vi "PubSubSync.vi"() -> ()   [LabVIEW 2025]
uses:
  libzmq-v143-mt-4_3_6/ctls/SocketType.ctl
  libzmq-v143-mt-4_3_6/ctls/SocketOption.ctl
  zeromq/Receive_string.vi
  zeromq/Send_string.vi
  zeromq/Context.lvclass
  libzmq-v143-mt-4_3_6/LibZMQ.lvlib
  zeromq/Socket.lvclass
panel:
  out "data 2":string
  out "data":string
  out "error out 2":errorcluster
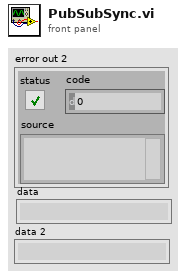
[diagram p1: front panel]
types:
  T1 = typedef "LibZMQ.lvlib/SocketOption.ctl" = enum8{"NONE", "ZMQ_HWM", "<2>", "ZMQ_SWAP", "ZMQ_AFFINITY", "ZMQ_ROUTING_ID", "ZMQ_SUBSCRIBE", "ZMQ_UNSUBSCRIBE", "ZMQ_RATE", "ZMQ_RECOVERY_IVL", "ZMQ_MCAST_LOOP", "ZMQ_SNDBUF", "ZMQ_RCVBUF", "ZMQ_RCVMORE", "ZMQ_FD", "ZMQ_EVENTS", "ZMQ_TYPE", "ZMQ_LINGER", "ZMQ_RECONNECT_IVL", "ZMQ_BACKLOG", "ZMQ_RECOVERY_IVL_MSEC", "ZMQ_RECONNECT_IVL_MAX", "ZMQ_MAXMSGSIZE", "ZMQ_SNDHWM", "ZMQ_RCVHWM", "ZMQ_MULTICAST_HOPS", "<26>", "ZMQ_RCVTIMEO", "ZMQ_SNDTIMEO", "<29>", "<30>", "ZMQ_IPV4ONLY", "ZMQ_LAST_ENDPOINT", "ZMQ_ROUTER_MANDATORY", "ZMQ_TCP_KEEPALIVE", "ZMQ_TCP_KEEPALIVE_CNT", "ZMQ_TCP_KEEPALIVE_IDLE", "ZMQ_TCP_KEEPALIVE_INTVL", "ZMQ_TCP_ACCEPT_FILTER", "ZMQ_IMMEDIATE", "ZMQ_XPUB_VERBOSE", "ZMQ_ROUTER_RAW", "ZMQ_IPV6", "ZMQ_MECHANISM", "ZMQ_PLAIN_SERVER", "ZMQ_PLAIN_USERNAME", "ZMQ_PLAIN_PASSWORD", "ZMQ_CURVE_SERVER", "ZMQ_CURVE_PUBLICKEY", "ZMQ_CURVE_SECRETKEY", "ZMQ_CURVE_SERVERKEY", "ZMQ_PROBE_ROUTER", "ZMQ_REQ_CORRELATE", "ZMQ_REQ_RELAXED", "ZMQ_CONFLATE", "ZMQ_ZAP_DOMAIN", "ZMQ_ROUTER_HANDOVER", "ZMQ_TOS", "ZMQ_IPC_FILTER_PID", "ZMQ_IPC_FILTER_UID", "ZMQ_IPC_FILTER_GID", "ZMQ_CONNECT_ROUTING_ID", "ZMQ_GSSAPI_SERVER", "ZMQ_GSSAPI_PRINCIPAL", "ZMQ_GSSAPI_SERVICE_PRINCIPAL", "ZMQ_GSSAPI_PLAINTEXT", "ZMQ_HANDSHAKE_IVL", "<67>", "ZMQ_SOCKS_PROXY", "ZMQ_XPUB_NODROP", "ZMQ_BLOCKY", "ZMQ_XPUB_MANUAL", "ZMQ_XPUB_WELCOME_MSG", "ZMQ_STREAM_NOTIFY", "ZMQ_INVERT_MATCHING", "ZMQ_HEARTBEAT_IVL", "ZMQ_HEARTBEAT_TTL", "ZMQ_HEARTBEAT_TIMEOUT", "ZMQ_XPUB_VERBOSER", "ZMQ_CONNECT_TIMEOUT", "ZMQ_TCP_MAXRT", "ZMQ_THREAD_SAFE", "<82>", "<83>", "ZMQ_MULTICAST_MAXTPDU", "ZMQ_VMCI_BUFFER_SIZE", "ZMQ_VMCI_BUFFER_MIN_SIZE", "ZMQ_VMCI_BUFFER_MAX_SIZE", "ZMQ_VMCI_CONNECT_TIMEOUT", "ZMQ_USE_FD", "ZMQ_GSSAPI_PRINCIPAL_NAMETYPE", "ZMQ_GSSAPI_SERVICE_PRINCIPAL_NAMETYPE", "ZMQ_BINDTODEVICE", "ZMQ_ZAP_ENFORCE_DOMAIN", "ZMQ_LOOPBACK_FASTPATH", "ZMQ_METADATA", "ZMQ_MULTICAST_LOOP", "ZMQ_ROUTER_NOTIFY"}
  T2 = typedef "LibZMQ.lvlib/SocketType.ctl" = enum8{"PAIR", "PUB", "SUB", "REQ", "REP", "DEALER", "ROUTER", "PULL", "PUSH", "XPUB", "XSUB", "STREAM"}
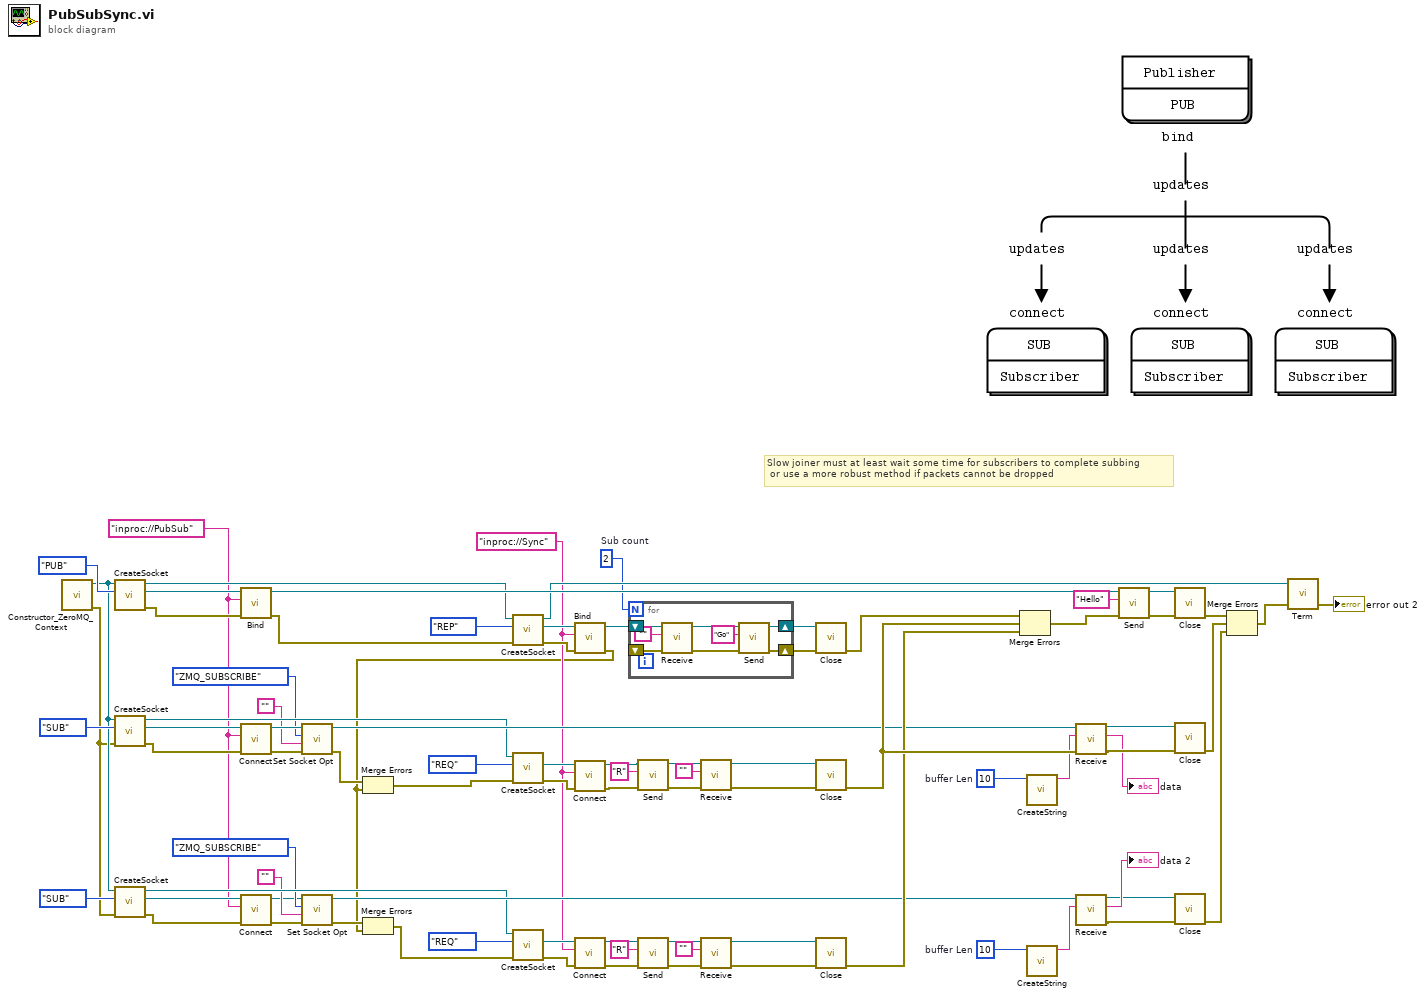
[diagram p0: block diagram]
diagram:
  w1 = "inproc://PubSub"
  w27 = 2  # Sub count
  w41 = "inproc://Sync"
  w61 = 10  # buffer Len
  w71 = 10  # buffer Len
  # "Slow joiner must at least wait some time for subscribers to complete subbing\n or use a more robust method if packets cannot be dropped"
  n1 = call "Constructor_ZeroMQ_Context.vi"() -> ("error out"=w16:errorcluster, "context out"=w57:refnum<class "Context.lvclass">)  [unwired: 10 in]
  n2 = call "CreateSocket.vi"("Socket Type"=SocketType."PUB", "context in"=w57) -> ("error out"=w25:errorcluster, "socket out"=w83:refnum<class "Socket.lvclass">, "context out"=w54:refnum<class "Context.lvclass">)  [unwired: 7 in]
  n3 = call "CreateSocket.vi"("error in"=w16, "Socket Type"=SocketType."SUB", "context in"=w57) -> ("error out"=w24:errorcluster, "socket out"=w81:refnum<class "Socket.lvclass">, "context out"=w46:refnum<class "Context.lvclass">)  [unwired: 6 in]
  n4 = call "CreateSocket.vi"("error in"=w16, "Socket Type"=SocketType."SUB", "context in"=w57) -> ("error out"=w23:errorcluster, "socket out"=w58:refnum<class "Socket.lvclass">, "context out"=w42:refnum<class "Context.lvclass">)  [unwired: 6 in]
  n5 = call "Bind.vi"("error in"=w25, "endpoint"=w1, "socket in"=w83) -> ("error out"=w15:errorcluster, "socket out"=w73:refnum<class "Socket.lvclass">)  [unwired: 7 in]
  n6 = call "Connect.vi"("error in"=w24, "endpoint"=w1, "socket in"=w81) -> ("error out"=w8:errorcluster, "socket out"=w9:refnum<class "Socket.lvclass">)  [unwired: 7 in]
  n7 = call "Connect.vi"("error in"=w23, "endpoint"=w1, "socket in"=w58) -> ("error out"=w3:errorcluster, "socket out"=w2:refnum<class "Socket.lvclass">)  [unwired: 7 in]
  n8 = call "Set Socket Opt.vi"("error in"=w8, "value"="", "Socket option"=SocketOption."ZMQ_SUBSCRIBE", "socket in"=w9) -> ("error out"=w14:errorcluster, "socket out"=w66:refnum<class "Socket.lvclass">)  [unwired: 6 in]
  n9 = call "Set Socket Opt.vi"("error in"=w3, "value"="", "Socket option"=SocketOption."ZMQ_SUBSCRIBE", "socket in"=w2) -> ("error out"=w12:errorcluster, "socket out"=w65:refnum<class "Socket.lvclass">)  [unwired: 6 in]
  n10 = call "CreateSocket.vi"("error in"=w15, "Socket Type"=SocketType."REP", "context in"=w54) -> ("error out"=w50:errorcluster, "socket out"=w51:refnum<class "Socket.lvclass">, "context out"=w53:refnum<class "Context.lvclass">)  [unwired: 6 in]
  n11 = call "Bind.vi"("error in"=w50, "endpoint"=w41, "socket in"=w51) -> ("error out"=w11:errorcluster, "socket out"=w37:refnum<class "Socket.lvclass">)  [unwired: 7 in]
  n12 = Merge Errors(w14, w11) -> (w13:errorcluster)
  n13 = Merge Errors(w12, w11) -> (w10:errorcluster)
  n14 = call "CreateSocket.vi"("error in"=w13, "Socket Type"=SocketType."REQ", "context in"=w46) -> ("error out"=w49:errorcluster, "socket out"=w48:refnum<class "Socket.lvclass">)  [unwired: 6 in, 1 out]
  n15 = call "CreateSocket.vi"("error in"=w10, "Socket Type"=SocketType."REQ", "context in"=w42) -> ("error out"=w43:errorcluster, "socket out"=w44:refnum<class "Socket.lvclass">)  [unwired: 6 in, 1 out]
  n16 = call "Connect.vi"("error in"=w49, "endpoint"=w41, "socket in"=w48) -> ("error out"=w35:errorcluster, "socket out"=w34:refnum<class "Socket.lvclass">)  [unwired: 7 in]
  n17 = call "Connect.vi"("error in"=w43, "endpoint"=w41, "socket in"=w44) -> ("error out"=w38:errorcluster, "socket out"=w40:refnum<class "Socket.lvclass">)  [unwired: 7 in]
  n18 = for {
    N: w27 -> [_]
    shift-right: [w88] -> w22
    shift-left: w37 -> [w93]
    shift-right: [w86] -> w21
    shift-left: _ -> [w92]
    n19 = call-poly "Receive.vi"("error in"=w92, "buf in"="", "socket in"=w93) -> ("error out"=w87:errorcluster, "socket out"=w89:refnum<class "Socket.lvclass">)  [unwired: 6 in, 1 out]
    n20 = call-poly "Send.vi"("error in"=w87, "data"="Go", "socket in"=w89) -> ("error out"=w86:errorcluster, "socket out"=w88:refnum<class "Socket.lvclass">)  [unwired: 7 in]
  }
  n21 = call-poly "Send.vi"("error in"=w35, "data"="R", "socket in"=w34) -> ("error out"=w32:errorcluster, "socket out"=w33:refnum<class "Socket.lvclass">)  [unwired: 7 in]
  n22 = call-poly "Send.vi"("error in"=w38, "data"="R", "socket in"=w40) -> ("error out"=w28:errorcluster, "socket out"=w29:refnum<class "Socket.lvclass">)  [unwired: 7 in]
  n23 = call-poly "Receive.vi"("error in"=w32, "buf in"="", "socket in"=w33) -> ("error out"=w19:errorcluster, "socket out"=w20:refnum<class "Socket.lvclass">)  [unwired: 6 in, 1 out]
  n24 = call-poly "Receive.vi"("error in"=w28, "buf in"="", "socket in"=w29) -> ("error out"=w17:errorcluster, "socket out"=w18:refnum<class "Socket.lvclass">)  [unwired: 6 in, 1 out]
  n25 = call "Close.vi"("error in"=w21, "socket"=w22) -> ("error out"=w26:errorcluster)  [unwired: 9 in]
  n26 = call "Close.vi"("error in"=w19, "socket"=w20) -> ("error out"=w85:errorcluster)  [unwired: 9 in]
  n27 = call "Close.vi"("error in"=w17, "socket"=w18) -> ("error out"=w84:errorcluster)  [unwired: 9 in]
  n28 = Merge Errors(w26, w85, w84) -> (w56:errorcluster)
  n29 = call "CreateString.vi"("length"=w71) -> ("string"=w72:string)  [unwired: 10 in]
  n30 = call "CreateString.vi"("length"=w61) -> ("string"=w60:string)  [unwired: 10 in]
  n31 = call-poly "Receive.vi"("error in"=w85, "buf in"=w72, "socket in"=w66) -> ("error out"=w69:errorcluster, "data"=→"data":string, "socket out"=w70:refnum<class "Socket.lvclass">)  [unwired: 6 in]
  n32 = call-poly "Receive.vi"("buf in"=w60, "socket in"=w65) -> ("error out"=w63:errorcluster, "data"=→"data 2":string, "socket out"=w62:refnum<class "Socket.lvclass">)  [unwired: 7 in]
  n33 = call-poly "Send.vi"("error in"=w56, "data"="Hello", "socket in"=w73) -> ("error out"=w75:errorcluster, "socket out"=w74:refnum<class "Socket.lvclass">)  [unwired: 7 in]
  n34 = call "Close.vi"("error in"=w75, "socket"=w74) -> ("error out"=w79:errorcluster)  [unwired: 9 in]
  n35 = call "Close.vi"("error in"=w69, "socket"=w70) -> ("error out"=w67:errorcluster)  [unwired: 9 in]
  n36 = call "Close.vi"("error in"=w63, "socket"=w62) -> ("error out"=w55:errorcluster)  [unwired: 9 in]
  n37 = Merge Errors(w79, w67, w55) -> (w78:errorcluster)
  n38 = call "Term.vi"("error in"=w78, "context in"=w53) -> ("error out"=→"error out 2":errorcluster)  [unwired: 3 in]
